vi "RSZVB Get Source Power Calibration Paramater Points.vi"(8 "error in (no error)":errorcluster {"code" format="%.0x"}, 9 "Calibration Index (1)":i32=1, 10 "Channel (1)":i32=1, 11 "VISA session":refnum<visa-resource-name>) -> (0 "error out":errorcluster {"code" format="%.0x"}, 2 "Points":i32, 3 "dup VISA session":refnum<visa-resource-name>)   [LabVIEW 2011]
doc: "This VI returns number of points of the active source and receiver power calibrations for channel <Ch>.\n\nRemote-control command(s):\nSOURce<Ch>:POWer<Pt>:CORRection:DATA:PARameter<Cal_index>? POIN"
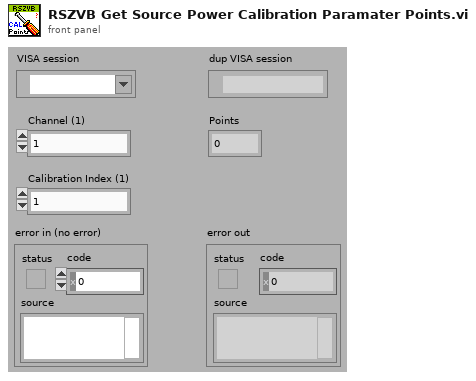
[diagram p1: front panel]
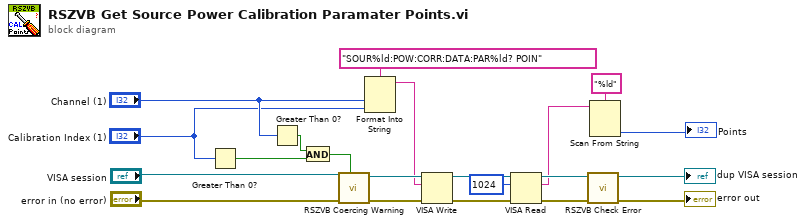
[diagram p0: block diagram]
diagram:
  n1 = Greater Than 0?(x="Calibration Index (1)") -> (x > 0?=w10:bool)
  n2 = Greater Than 0?(x="Channel (1)") -> (x > 0?=w11:bool)
  n3 = And(x=w11, y=w10) -> (x .and. y?=w12:bool)
  n4 = call "RSZVB Coercing Warning.vi"("In Range?"=w12, "error in (no error)"="error in (no error)", "VISA session"="VISA session") -> ("error out"=w15:errorcluster, "dup VISA session"=w16:refnum<visa-resource-name>)  [unwired: 7 in]
  n5 = Format Into String(format string="SOUR%ld:POW:CORR:DATA:PAR%ld? POIN", "Channel (1)", "Calibration Index (1)") -> (resulting string=w13:string)  [unwired: 2 in, 1 out]
  n6 = VISA Write(VISA resource name=w16, write buffer=w13, error in (no error)=w15) -> (VISA resource name out=w20:refnum<visa-resource-name>, error out=w21:errorcluster)  [unwired: 1 out]
  n7 = VISA Read(VISA resource name=w20, byte count=u32 1024, error in (no error)=w21) -> (VISA resource name out=w17:refnum<visa-resource-name>, read buffer=w8:string, error out=w18:errorcluster)  [unwired: 1 out]
  n8 = call "RSZVB Check Error.vi"("error in (no error)"=w18, "VISA session"=w17) -> ("error out"=→"error out":errorcluster, "dup VISA session"=→"dup VISA session":refnum<visa-resource-name>)  [unwired: 8 in]
  n9 = Scan From String(format string="%ld", input string=w8) -> (output 1=→"Points":i32)  [unwired: 3 in, 3 out]
